vi "Initialize.vi"(8 "error in":errorcluster, 9 "Set All to Input?":bool=TRUE, 10 "baud rate":u32=57600, 11 "comport":refnum<visa-resource-name>="COM20") -> (0 "error out":errorcluster={"status"=TRUE, "code"=-1073807339, "source"="VISA Read in FirmataClient.lvlib:Initialize.vi"}, 1 "Initialize Was Successful":bool, 2 "result":string, 3 "comport out":refnum<visa-resource-name>)   [LabVIEW 2020, in "FirmataClient.lvlib"]
doc: "Initializes the target device. Using an opinionated configuration for the pins of the UUT device"
uses:
  FirmataClient.lvlib
  controls/FGV-Mode.ctl
  controls/FirmataPinModes.ctl
  <vilib>/regexp/Match Regular Expression.xnode
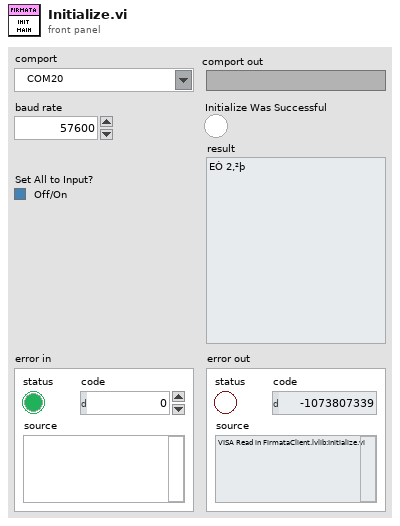
[diagram p1: front panel]
types:
  T1 = typedef "FirmataClient.lvlib/FGV-Mode.ctl" = enum16{"Load Comport", "Load Board Capabilities", "Read"}
  T2 = typedef "FirmataClient.lvlib/FirmataPinModes.ctl" = enum16{"DigitalInput", "DigitalOutput", "AnalogInput", "PWM", "Servo", "Shift", "I2C", "OneWire", "Stepper", "Encoder", "Serial", "InputPullup", "Extended.SPI", "Extended.Sonar", "Extended.Tone", "Extended.DHT"}
  T3 = typedef "FirmataClient.lvlib/FirmataProtocolConstants.ctl" = u16
  T4 = typedef "FirmataClient.lvlib/PinModesListData.ctl" = cluster{"DigitalInputMode":T5, "DigitalOutputMode":T5, "AnalogInputMode":T5, "PWMMode":T5, "ServoMode":T5, "ShiftMode":T5, "I2CMode":T5, "OneWireMode":T5, "StepperMode":T5, "EncoderMode":T5, "SerialMode":T5, "InputPullupMode":T5, "Ext.SPIMode":T5, "Ext.SonarMode":T5, "Ext.ToneMode":T5, "Ext.DHTMode":T5, "Index":cluster{"DigitalIndex":u16, "AnalogIndex":dbl}}
  T5 = typedef "FirmataClient.lvlib/PinModeData.ctl" = cluster{"Resolution":u8, "btn":bool, "PinMode":T2}
  T6 = typedef "FirmataProtocolConstants.ctl" = u16
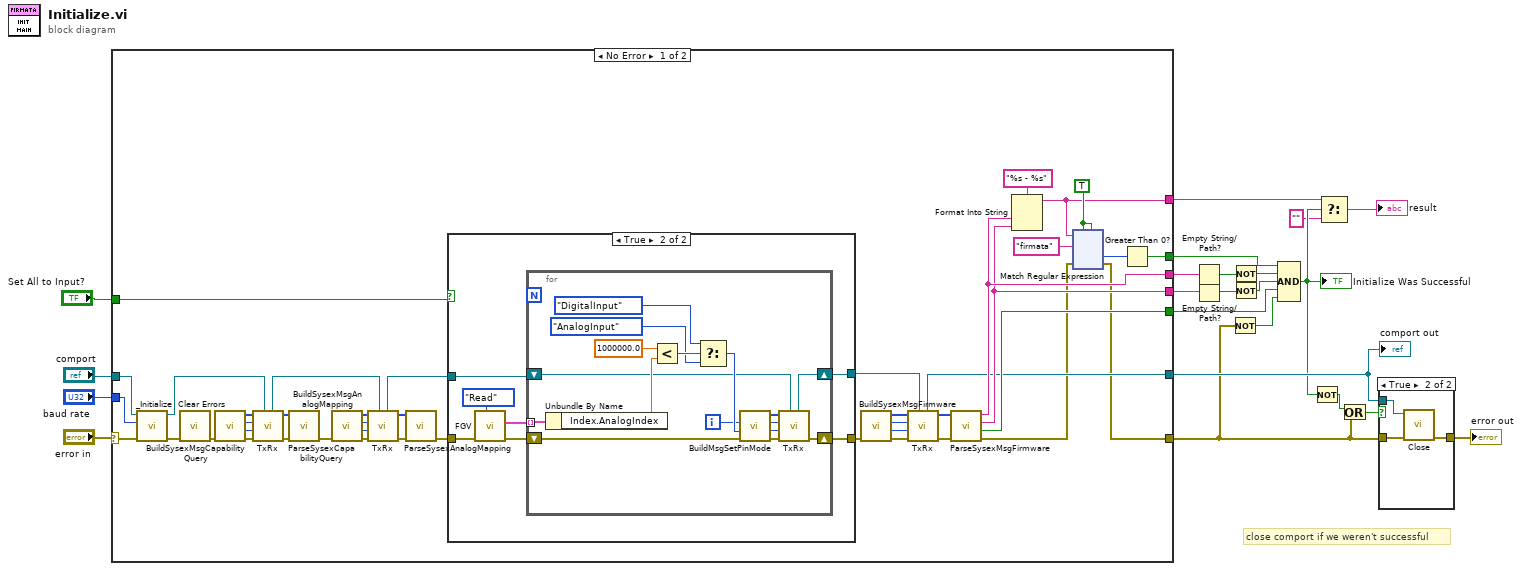
[diagram p0: block diagram]
diagram:
  # "close comport if we weren't successful"
  n1 = case shown="No Error" "error in" {
    selector: "error in" -> [w62 w206]
    tunnel: [w23 w206] -> w9
    tunnel: "comport" -> [w61 w205]
    tunnel: "baud rate" -> [w60 _]
    tunnel: [w59 _] -> w16
    tunnel: [w58 _] -> w22
    tunnel: [w57 _] -> w21
    tunnel: [w32 w205] -> w10
    tunnel: [w27 _] -> w6
    tunnel: [w26 _] -> w4
    tunnel: "Set All to Input?" -> [w25 _]
    frame No Error {
      w29 = TRUE ("ignore case? (F)")
      n2 = call "_Initialize.vi"("error in"=w62, "baud rate"=w60, "comport"=w61) -> ("error out"=w65:errorcluster, "comport out"=w46:refnum<visa-resource-name>)  [unwired: 4 in, 3 out]
      n3 = call <vilib>:"Clear Errors.vi"("error in (no error)"=w65) -> ("error out"=w47:errorcluster)  [unwired: 5 in, 1 out]
      n4 = call "BuildSysexMsgCapabilityQuery.vi"("error in"=w47) -> ("error out"=w56:errorcluster, "ReplyLength"=w41:i32, "ReplyFirstByte"=w42:T3, "GetCapabilitiesMessage"=w43:u8[])  [unwired: 7 in]
      n5 = call "TxRx.vi"("comport in"=w46, "error in"=w56, "Expected Reply Length"=w41, "ReplyFirstByte"=w42, "MessageToSend"=w43) -> ("error out"=w55:errorcluster, "ReceivedMessage"=w40:u8[], "comport out"=w45:refnum<visa-resource-name>)  [unwired: 2 in, 2 out]
      n6 = call "ParseSysexCapabilityQuery.vi"("error in"=w55, "Sysex Message"=w40) -> ("error out"=w52:errorcluster)  [unwired: 7 in, 2 out]
      n7 = call "BuildSysexMsgAnalogMapping.vi"("error in"=w52) -> ("error out"=w53:errorcluster, "ReplyLength"=w49:i32, "ReplyFirstByte"=w38:T3, "GetAnalogMappingMessage"=w39:u8[])  [unwired: 7 in]
      n8 = call "TxRx.vi"("comport in"=w45, "error in"=w53, "Expected Reply Length"=w49, "ReplyFirstByte"=w38, "MessageToSend"=w39) -> ("error out"=w54:errorcluster, "ReceivedMessage"=w37:u8[], "comport out"=w44:refnum<visa-resource-name>)  [unwired: 2 in, 2 out]
      n9 = call "ParseSysexAnalogMapping.vi"("error in"=w54, "Sysex Message"=w37) -> ("error out"=w51:errorcluster)  [unwired: 7 in, 2 out]
      n10 = case shown="True" w25 {
        tunnel: w51 -> [w181 w187]
        tunnel: [w181 w185] -> w50
        tunnel: w44 -> [w180 w183]
        tunnel: [w180 w182] -> w36
        frame False {
        }
        frame True {
          n11 = call "FGV.vi"("Mode"=FGV-Mode."Read", "error in"=w187) -> ("error out"=w186:errorcluster, "Board Pins Out"=w184:T4[])  [unwired: 7 in, 1 out]
          n12 = for {
            shift-right: [w202] -> w185
            shift-left: w186 -> [w203]
            tunnel: w184 -> [w201] mode=indexing
            shift-right: [w191] -> w182
            shift-left: w183 -> [w192]
            i -> [w193]
            n13 = Unbundle By Name(w201) -> ("Index.AnalogIndex"=w200:dbl)
            n14 = Less?(x=1000000.0, y=w200) -> (x < y?=w198:bool)
            n15 = Select(t=FirmataPinModes."DigitalInput" ("FirmataPinModes"), s=w198, f=FirmataPinModes."AnalogInput" ("FirmataPinModes")) -> (s? t:f=w194:T2)
            n16 = call "BuildMsgSetPinMode.vi"("error in"=w203, "Pin Mode"=w194, "Pin Index"=w193) -> ("error out"=w204:errorcluster, "ReplyLength"=w197:i32, "ReplyFirstByte"=w189:T3, "SetPinModeMessage"=w190:u8[])  [unwired: 5 in]
            n17 = call "TxRx.vi"("comport in"=w192, "error in"=w204, "Expected Reply Length"=w197, "ReplyFirstByte"=w189, "MessageToSend"=w190) -> ("error out"=w202:errorcluster, "comport out"=w191:refnum<visa-resource-name>)  [unwired: 2 in, 3 out]
          }
        }
      }
      n18 = call "BuildSysexMsgFirmware.vi"("error in"=w50) -> ("error out"=w63:errorcluster, "ReplyLength"=w48:i32, "ReplyFirstByte"=w34:T6, "GetFirmwareMessage"=w35:u8[])  [unwired: 7 in]
      n19 = call "TxRx.vi"("comport in"=w36, "error in"=w63, "Expected Reply Length"=w48, "ReplyFirstByte"=w34, "MessageToSend"=w35) -> ("error out"=w64:errorcluster, "ReceivedMessage"=w33:u8[], "comport out"=w32:refnum<visa-resource-name>)  [unwired: 2 in, 2 out]
      n20 = call "ParseSysexMsgFirmware.vi"("error in"=w64, "Sysex Message"=w33) -> ("error out"=w24:errorcluster, "IsValidSysex"=w59:bool, "FirmataFirmwareVersion"=w57:string, "FirmataFirmwareName"=w58:string)  [unwired: 6 in]
      n21 = Format Into String(format string="%s - %s", w58, w57) -> (resulting string=w26:string)  [unwired: 2 in, 1 out]
      n22 = xnode "Match Regular Expression"("input string"=w26, "regular expression"="firmata", "error in"=w24, "ignore case? (F)"=w29, "multiline? (F)"=w29) -> ("offset past match"=w31:i32, "error out"=w23:errorcluster)  [unwired: 1 in, 3 out]
      n23 = Greater Than 0?(x=w31) -> (x > 0?=w27:bool)
    }
    frame Error {
    }
  }
  "comport out" <- w10
  n24 = Empty String/Path?(string/path=w22) -> (empty?=w20:bool)
  n25 = Empty String/Path?(string/path=w21) -> (empty?=w19:bool)
  n26 = Not(x=w9) -> (.not. x?=w15:bool)
  n27 = Not(x=w20) -> (.not. x?=w18:bool)
  n28 = Not(x=w19) -> (.not. x?=w17:bool)
  n29 = Compound Arithmetic op=AND(w6, w18, w17, w16, w15) -> (w5:bool)
  "Initialize Was Successful" <- w5
  n30 = Not(x=w5) -> (.not. x?=w7:bool)
  n31 = Select(t=w4, s=w5, f="") -> (s? t:f=→"result":string)
  n32 = Or(x=w7, y=w9) -> (x .or. y?=w8:bool)
  n33 = case shown="True" w8 {
    tunnel: w9 -> [w207 w210]
    tunnel: [w207 w209] -> w11
    tunnel: w10 -> [_ w208]
    frame False {
    }
    frame True {
      n34 = call "Close.vi"("error in"=w210, "VISA resource name"=w208) -> ("error out"=w209:errorcluster)  [unwired: 9 in]
    }
  }
  "error out" <- w11
